vi "UpdateTable.vi"(8 "error in (no error)":errorcluster, 11 "HealthCheck in":refnum<class "HealthCheck.lvclass">) -> (0 "error out":errorcluster, 3 "HealthCheck out":refnum<class "HealthCheck.lvclass">)   [LabVIEW 2018, in "HealthCheck.lvclass"]
uses:
  HealthCheck.lvclass
  HealthCheck.lvclass/HealthCheck.ctl
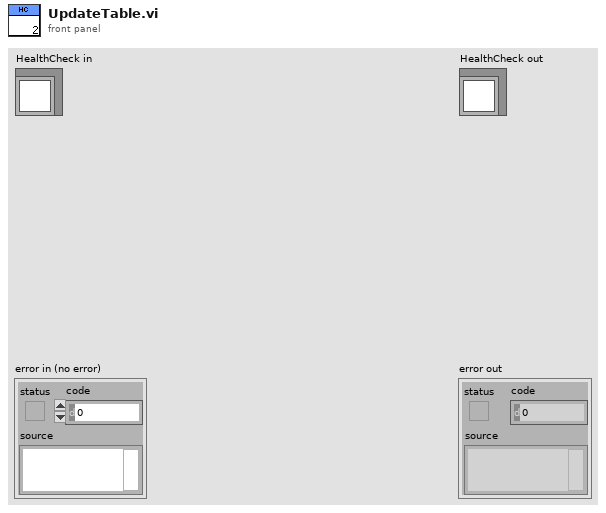
[diagram p1: front panel]
types:
  T1 = typedef "HealthCheck.lvclass/DataEntry_TypeDef.ctl" = cluster{"Data Name":string, "Units":string, "Minimum Value":string, "Maximum Value":string, "Actual Value":string, "Precision":i16}
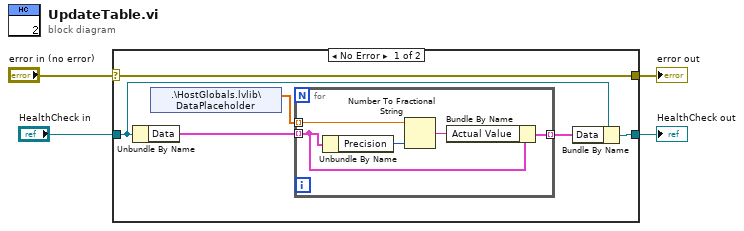
[diagram p0: block diagram]
diagram:
  n1 = case shown="No Error" "error in (no error)" {
    selector: "error in (no error)" -> [w10 w17]
    tunnel: [w10 w17] -> w3
    tunnel: [w7 w16] -> w1
    tunnel: "HealthCheck in" -> [w6 w16]
    frame No Error {
      n2 = Unbundle By Name(w6) -> ("Data"=w9:T1[])
      n3 = shared-variable ".\\HostGlobals.lvlib\\DataPlaceholder"() -> (w5:dbl[])  [unwired: 1 in, 1 out]
      n4 = for {
        tunnel: w9 -> [w12] mode=indexing
        tunnel: [w15] -> w8 mode=indexing
        tunnel: w5 -> [w14] mode=indexing
        n5 = Unbundle By Name(w12) -> ("Precision"=w11:i16)
        n6 = Number To Fractional String(number=w14, precision (6)=w11) -> (F-format string=w13:string)  [unwired: 2 in]
        n7 = Bundle By Name(cluster=w12, "Actual Value"=w13) -> (w15:T1)
      }
      n8 = Bundle By Name(cluster=w6, "Data"=w8) -> (w7:refnum<class "HealthCheck.lvclass">)
    }
    frame Error {
    }
  }
  "error out" <- w3
  "HealthCheck out" <- w1
